vi "Brass_4_Int.vi"() -> ()   [LabVIEW 2015]
uses:
  TypeDefs Host/Keyboard.ctl
  <vilib>/Platform/TimedLoop/XDataNode/timing_clust.ctl
  <vilib>/Platform/TimedLoop/XDataNode/nitl_modes.ctl
  <vilib>/Platform/TimedLoop/XDataNode/wakeup.ctl
  TypeDefs Host/Scales.ctl
  <vilib>/rvi/Emulation/niFpgaGetClockAttributes.vi
  <vilib>/rvi/Emulation/niFpgaSctlEmulationGetInTimedLoop.vi
  <vilib>/rvi/Emulation/niFpgaEmulationReportErrorSimple.vi
  <vilib>/rvi/Emulation/niFpgaCriticalErrorInLSC.vi
  <vilib>/rvi/Emulation/niFpgaEmulationIsFPGAContextNoSignature.vi
  <vilib>/rvi/errors/niFpgaSetErrorForExecOnDevCompSimple.vi
  <vilib>/rvi/eio/common/nirviEmuReportErrorAndStop.vi
  <vilib>/rvi/DataTransferAndStorage/Container/Common/niFpgaContainerGetUniqueNameForEmu.vi
  <vilib>/rvi/FIFO/Fifo_Resource/nirvififoEmulationSetSize.vi
  <vilib>/rvi/FIFO/Fifo_Resource/nirviFifoEmulationQueueMgr.vi
  <instcachedir>/0/nirviFifoEmulationQueueMgr_E5CAEC123FF24DC58D834DCA3CDAA9B5.lvgen/nirviFifoEmulationQueueMgr_E5CAEC123FF24DC58D834DCA3CDAA9B5_001.vi
  <vilib>/rvi/FIFO/Fifo_Resource/nirvififoEmulationDetermineInputValidOut.vi
  <vilib>/rvi/FIFO/Fifo_Resource/nirvififoEmulationCreateLock.vi
  <vilib>/rvi/Emulation/niFpgaProcessEmulError.vi
  <vilib>/rvi/FIFO/Fifo_Resource/nirvififoEmulationObtainLock.vi
  <vilib>/rvi/FIFO/Fifo_Resource/nirvififoEmulationReleaseLock.vi
  <vilib>/rvi/occurrence/nirviWaitOnOccurrenceBase.vi
  <vilib>/rvi/errors/nirviReportUnexpectedCaseInternalError.vi
  <vilib>/rvi/errors/nirviReportUnexpectedCaseInternalError (U32).vi
  <vilib>/Utility/error.llb/Clear Errors.vi
  <vilib>/rvi/eio/common/nirviEmuTemplateMethod_errors.vi
  <vilib>/Platform/TimedLoop/XDataNode/XDataNode.xnode
  <vilib>/rvi/DataTransferAndStorage/Container/XNode/niFpgaContainer.xnode
  <vilib>/rvi/FIFO/Fifo_Resource/nirvififoEmulationWrite.vi
  <vilib>/rvi/FIFO/Fifo_Resource/nirvififoEmulationRead.vi
  <vilib>/eio/EIONode/EIONode.xnode
  <vilib>/Platform/TimedLoop/XDataNode/XDNodeRunTimeDep.lvlib
panel:
  in  "M LFO":fxp<+,32,32>
  in  "Keyboard 2":T1
  in  "Keyboard":T1
  in  "1/2":bool
  in  "Scale":i8
  in  "Levels":u8
  in  "Delay?":bool
  in  "1/Attack":fxp<+,16,0>
  in  "1/Decay":fxp<+,16,0>
  in  "Sustain":fxp<+,16,0>
  in  "S/R":fxp<+,16,0>
  in  "Amount":fxp<+,8,0>
  in  "Gate":bool
  out "VCA Out":i16
  in  "Transfer":bool
  # "VCO"
  # "VCA"
  # "Rep"
  # "Interf"
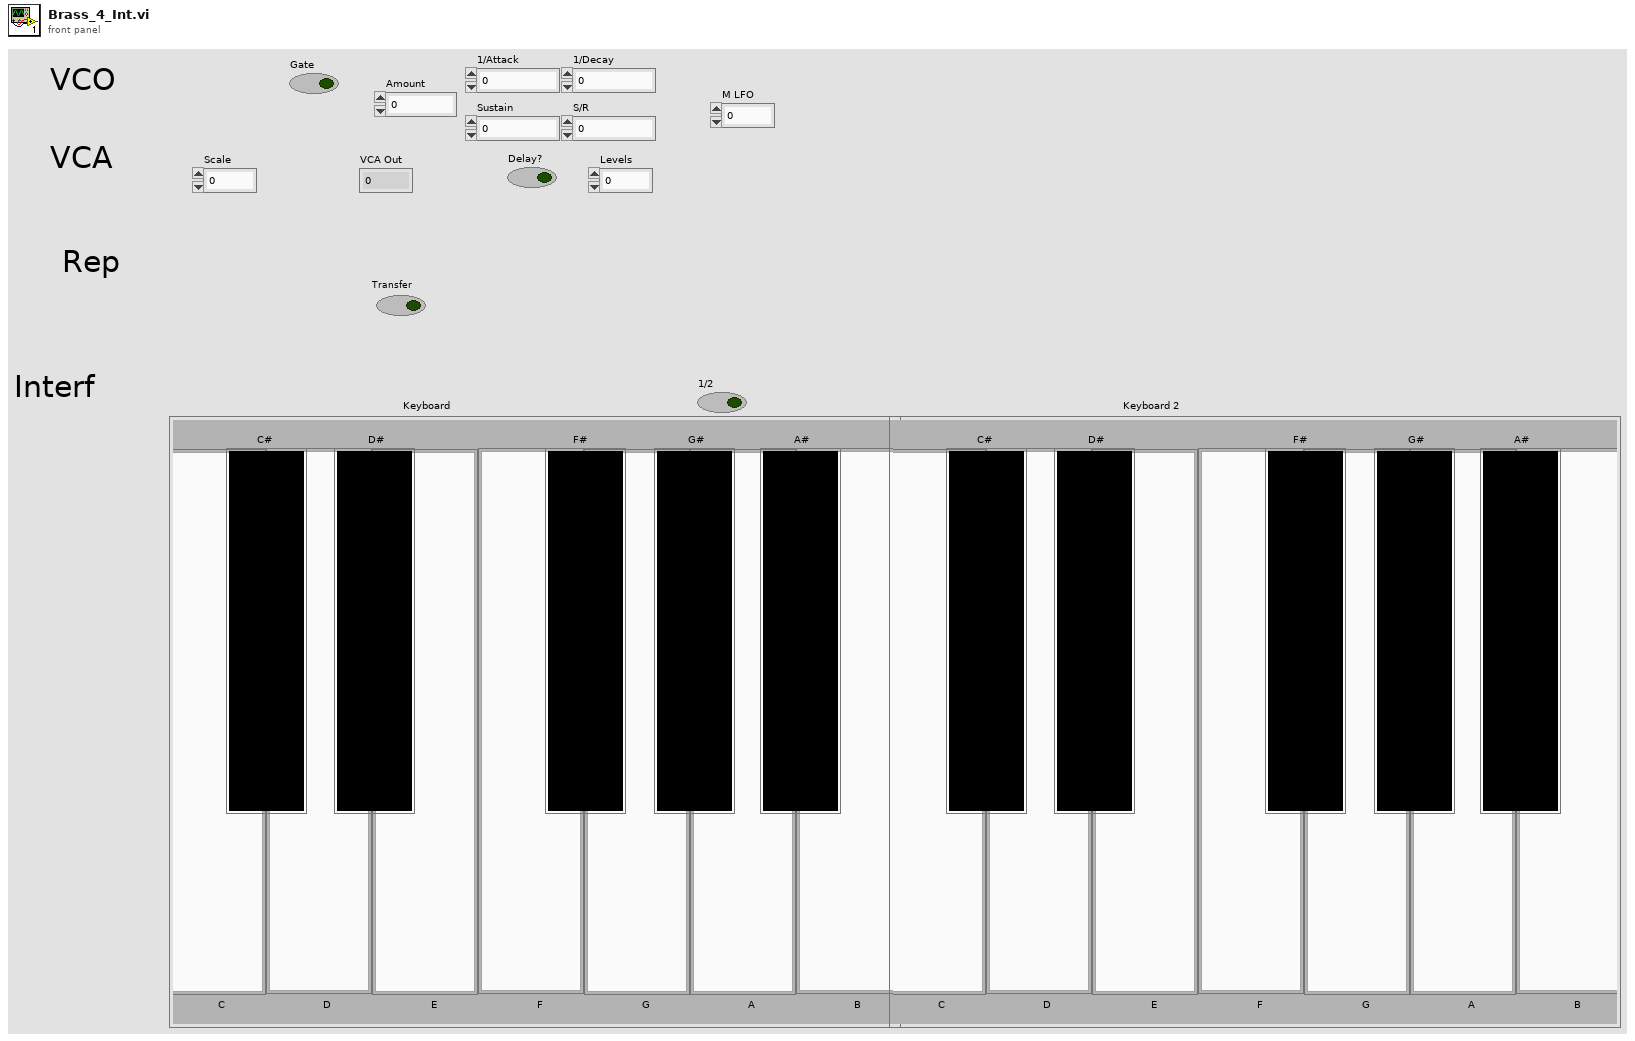
[diagram p1: front panel]
types:
  T1 = typedef "Keyboard.ctl" = cluster{"C":bool, "C#":bool, "D":bool, "D#":bool, "E":bool, "F":bool, "F#":bool, "G":bool, "G#":bool, "A":bool, "A#":bool, "B":bool}
  T2 = typedef "XDNodeRunTimeDep.lvlib/timing_clust.ctl" = cluster{"Expected End [f-1]":u64, "Actual End [f-1]":u64, "Finished Late? [f-1]":bool, "Expected End [i-1]":u64, "Actual End [i-1]":u64, "Finished Late? [i-1]":bool, "Expected Start [i]":u64, "Actual Start [i]":u64, "Expected Start [f]":u64, "Actual Start [f]":u64, "Source Name":string, "Structure Name":string, "Period":i64, "Deadline":i64, "Offset":i64, "Start":i64, "Priority":i32, "Timeout":i32, "Mode":T3, "Wakeup Reason":T4, "Error":errorcluster, "Source Type":string, "Secondary Source Type":string, "Global End Time":u64, "Global Start Time":u64, "Frame Duration":u64, "Iteration Duration":u64, "Assigned CPU":i32, "I/O Scan Engine Mode":u32}
  T3 = typedef "XDNodeRunTimeDep.lvlib/nitl_modes.ctl" = enum32{"No Change", "Process missed periods, maintain original phase", "Discard missed periods, maintain original phase", "Process missed periods, ignore original phase", "Discard missed periods, ignore original phase"}
  T4 = typedef "XDNodeRunTimeDep.lvlib/wakeup.ctl" = enum32{"Normal", "Aborted", "Asynchronous wakeup", "Timing source error", "Timed loop error", "Timeout"}
  T5 = typedef "Scales.ctl" = enum16{"ALL", "DO", "RE"}
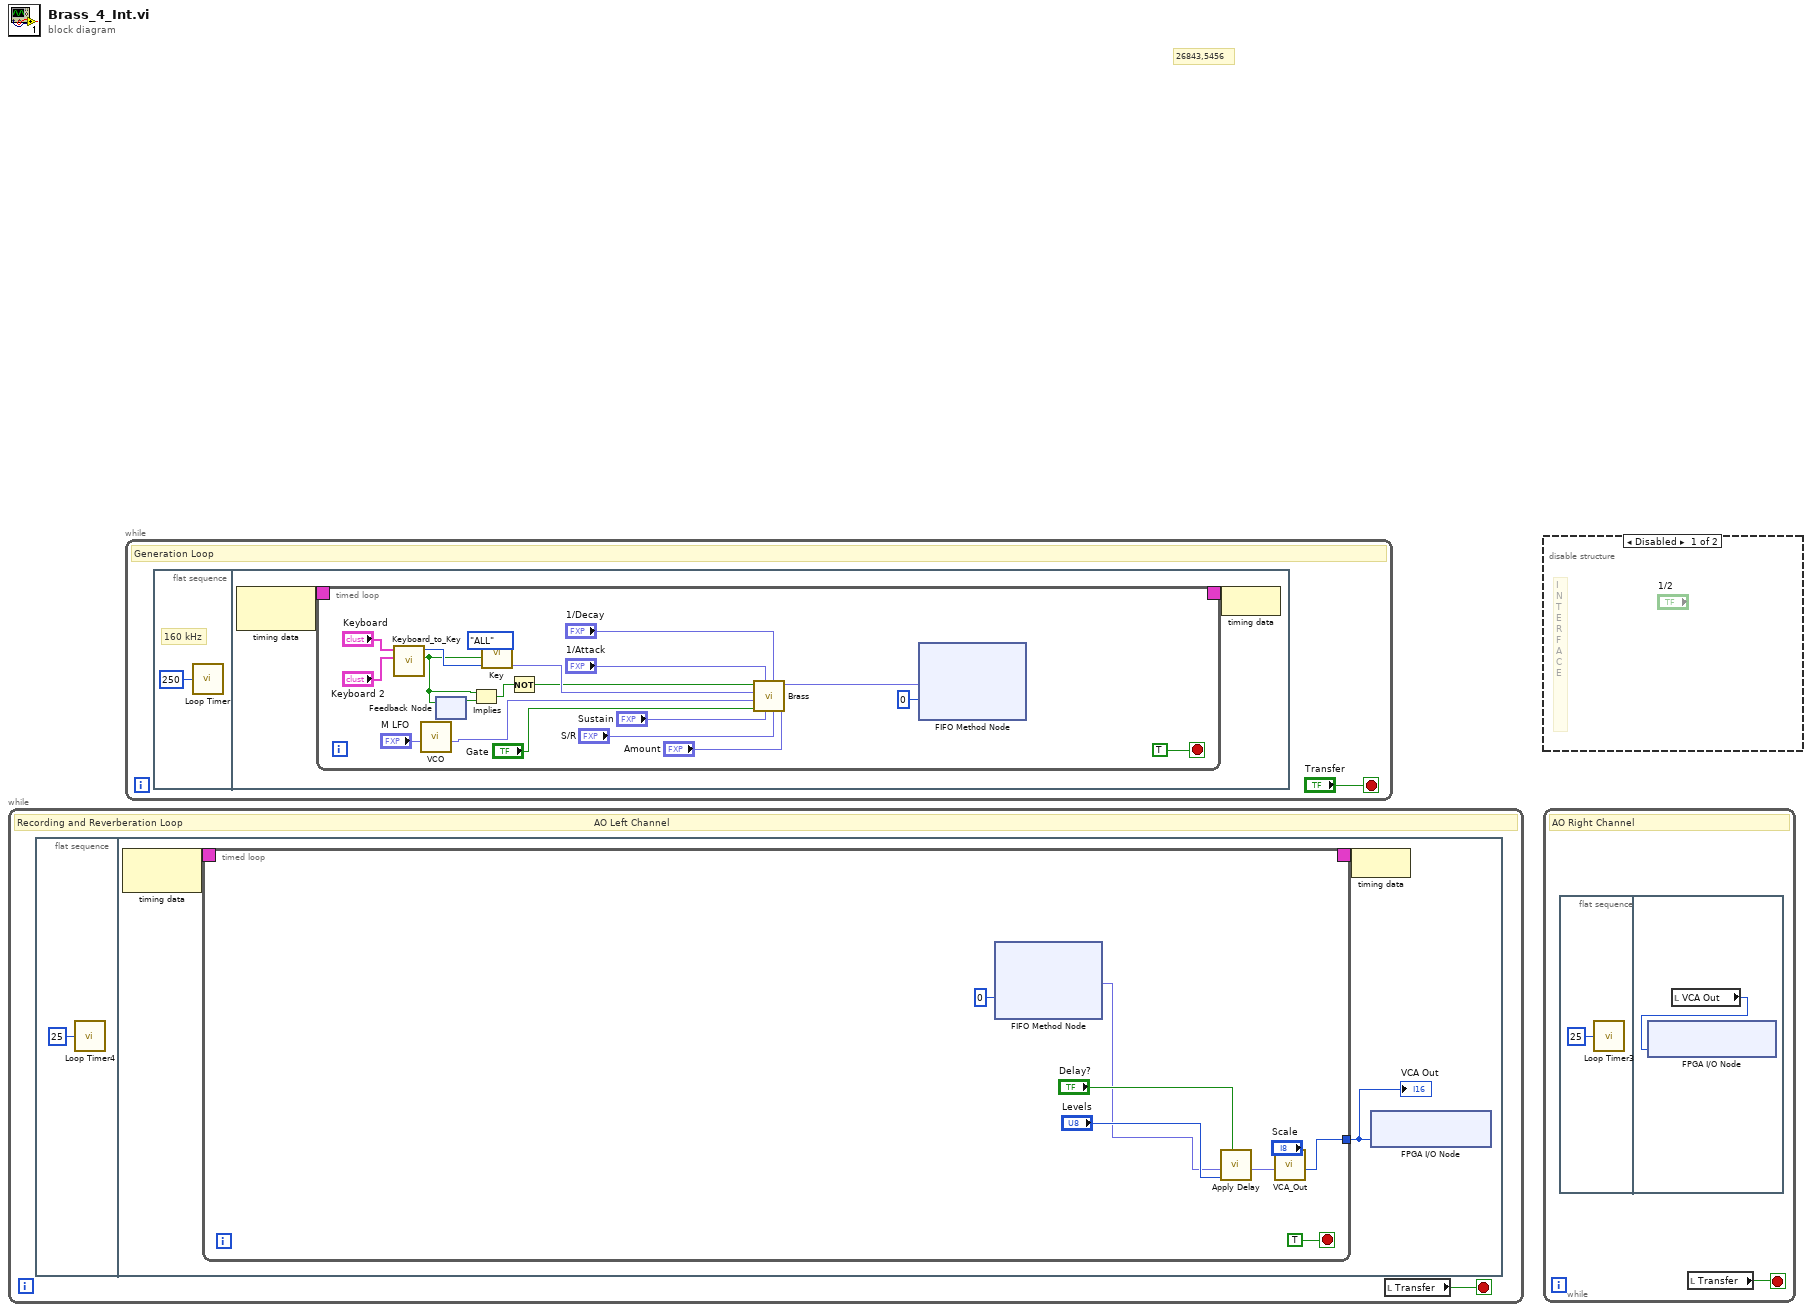
[diagram p0: block diagram]
diagram:
  # "26843,5456"
  n1 = while {
    stop <- w1 stop-if-true
    # "Recording and Reverberation Loop                                                                                                                                         AO Left Channel"
    n2 = flat-sequence {
      frame #0 {
        n3 = call "Loop Timer4"("Count(uSec)"=u8 25) -> ()  [unwired: 1 out]
      }
      frame #1 {
        n4 = node-c288() -> (w5:T2)  [unwired: 1 in]
        n5 = timed-loop {
          timing: w5 -> [_]
          timing-out: [_] -> w4
          tunnel: [w7] -> w3
          stop <- TRUE stop-if-true
          n6 = xnode ("FIFO Method Node")("Timeout"=0) -> ("Element"=w6:fxp<+/-,8,8>)  [unwired: 1 in, 2 out]
          n7 = call "Apply Delay.vi"("Delay?"="Delay?", "Levels"="Levels", "Element in"=w6) -> ("Element out"=w12:fxp<+/-,8,8>)  [unwired: 8 in]
          n8 = call "VCA_Out.vi"("Scale"="Scale", "Sample In"=w12) -> ("Sample Out"=w7:i16)  [unwired: 9 in]
        }
        "VCA Out" <- w3
        n9 = node-c288(w4) -> ()
        n10 = xnode "FPGA I/O Node"("AudioOut/Left"=w3) -> ()  [unwired: 1 in, 1 out]
      }
    }
    n11 = local read "Transfer"() -> (w1:bool)
  }
  n12 = while {
    stop <- "Transfer" stop-if-true
    # "Generation Loop"
    n13 = flat-sequence {
      frame #0 {
        # "160 kHz"
        n14 = call "Loop Timer"("Count(Ticks)"=u8 250) -> ()  [unwired: 1 out]
      }
      frame #1 {
        n15 = node-c288() -> (w21:T2)  [unwired: 1 in]
        n16 = timed-loop {
          timing: w21 -> [_]
          timing-out: [_] -> w20
          stop <- TRUE stop-if-true
          n17 = call "Keyboard_to_Key.vi"("Keyboard 2"="Keyboard 2", "Keyboard"="Keyboard") -> ("Key pressed?"=w27:bool, "Key index"=w33:u8)  [unwired: 8 in]
          n18 = call "VCO.vi"("M"="M LFO") -> ("Sine Sample"=w23:fxp<+/-,8,8>)  [unwired: 10 in]
          n19 = feedback-in #1(w27) -> ()
          n20 = feedback #1() -> (w28:bool)  [unwired: 1 in]
          n21 = Implies(1:w28, 2:w27) -> (0:w26:bool)
          n22 = call "Key.vi"("Scale"=Scales."ALL", "Key"=w33, "Enable"=w27) -> ("M"=w29:fxp<+,32,32>)  [unwired: 7 in, 1 out]
          n23 = Not(x=w26) -> (.not. x?=w25:bool)
          n24 = call "Brass.vi"("Amount"="Amount", "S/R"="S/R", "1/Decay"="1/Decay", "Sustain"="Sustain", "1/Attack"="1/Attack", "Gate"="Gate", "LFO"=w23, "M"=w29, "Trigger"=w25) -> ("Brass Out"=w24:fxp<+/-,8,8>)  [unwired: 2 in]
          n25 = xnode ("FIFO Method Node")("Element"=w24, "Timeout"=0) -> ()  [unwired: 1 in, 2 out]
        }
        n26 = node-c288(w20) -> ()
      }
    }
  }
  n27 = disable-structure shown="Disabled" {
    frame Disabled {
      # "I\nN\nT\nE\nR\nF\nA\nC\nE"
    }
    frame Enabled {
    }
  }
  n28 = while {
    stop <- w46 stop-if-true
    # "AO Right Channel"
    n29 = flat-sequence {
      frame #0 {
        n30 = call "Loop Timer3"("Count(uSec)"=u8 25) -> ()  [unwired: 1 out]
      }
      frame #1 {
        n31 = local read "VCA Out"() -> (w48:i16)
        n32 = xnode "FPGA I/O Node"("AudioOut/Right"=w48) -> ()  [unwired: 1 in, 1 out]
      }
    }
    n33 = local read "Transfer"() -> (w46:bool)
  }
